vi "Debug Dequeuer.vi"() -> ()   [LabVIEW 2013]
panel:
  out "Waveform Chart":dbl[][](graph)
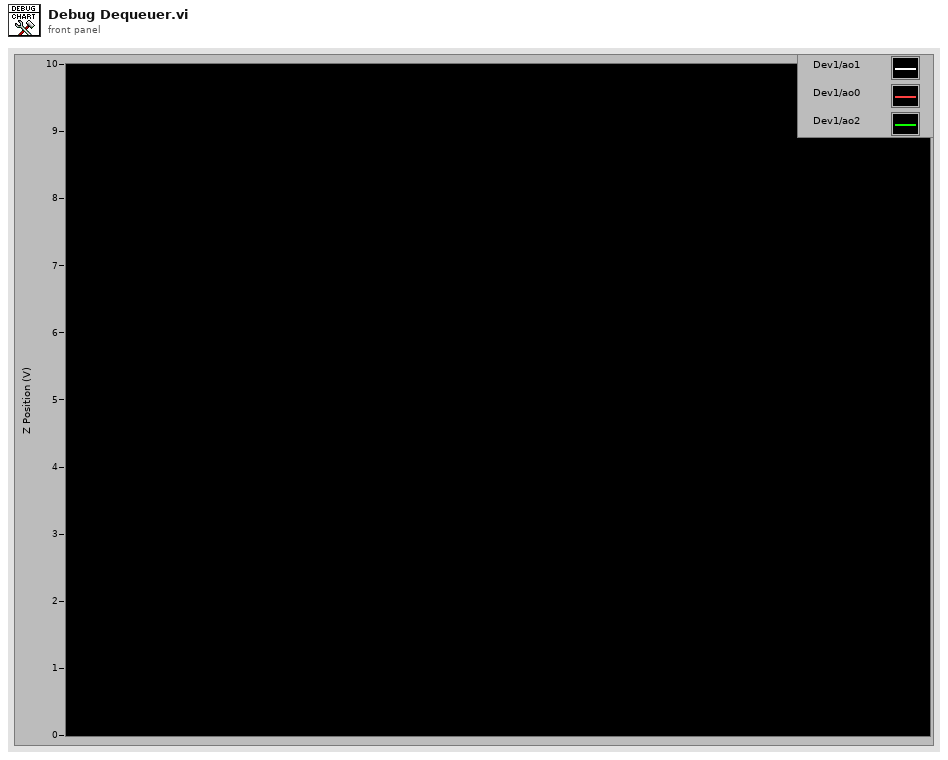
[diagram p1: front panel]
types:
  T1 = typedef "Sidecar Debug Queue.ctl" = refnum<queue>
  T2 = typedef "Experimental Configuration.ctl" = cluster{"Output Waveforms":waveform(dbl)[], "Output Channels":string, "Input Channels":string, "Post-Hook Occurence":refnum<k4>}
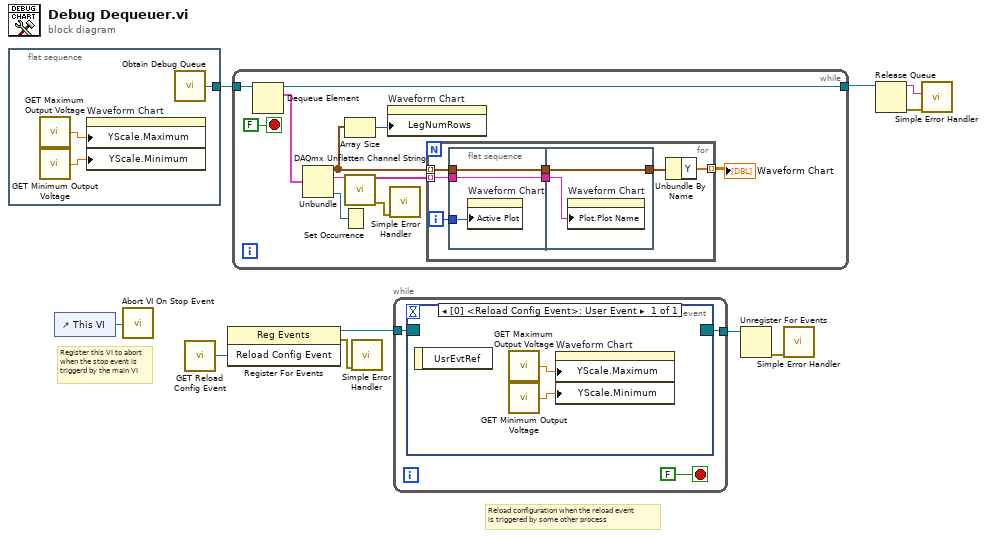
[diagram p0: block diagram]
diagram:
  # "Reload configuration when the reload event\nis triggered by some other process"
  # "Register this VI to abort\nwhen the stop event is\ntriggerd by the main VI"
  n1 = flat-sequence {
    tunnel: [w13] -> w10
    frame #0 {
      n2 = call "GET Maximum Output Voltage.vi"() -> ("Maximum Output Voltage"=w12:dbl)
      n3 = call "GET Minimum Output Voltage.vi"() -> ("Minimum Output Voltage"=w11:dbl)
      n4 = property on="Waveform Chart" class="WFChart (strict)"("YScale.Maximum"=w12, "YScale.Minimum"=w11) -> ()  [unwired: 2 in, 2 out]
      n5 = call "Obtain Debug Queue.vi"() -> ("Debug Queue"=w13:T1)
    }
  }
  n6 = control-ref of="This VI"() -> (w6:refnum<vi>)
  n7 = call "Abort VI On Stop Event.vi"("VI Reference"=w6) -> ()
  n8 = call "GET Reload Config Event.vi"() -> ("Reload Config Event"=w5:refnum<user-event>)
  n9 = register-events(w5) -> (reference out=w4:refnum<event-registration>, error out=w3:errorcluster)  [unwired: 2 in]
  n10 = while {
    tunnel: w10 -> [w23]
    tunnel: [w22] -> w9
    stop <- FALSE stop-if-true
    n11 = Dequeue Element(queue=w23) -> (queue out=w22:T1, element=w21:T2)  [unwired: 2 in, 2 out]
    n12 = Unbundle(w21) -> ("Output Waveforms"=w19:waveform(dbl)[], "Output Channels"=w17:string, "Post-Hook Occurence"=w20:refnum<k4>)  [unwired: 1 out]
    n13 = Set Occurrence(w20) -> ()
    n14 = Array Size(array=w19) -> (size(s)=w18:i32)
    n15 = call <vilib>:"DAQmx Unflatten Channel String.vi"("names in"=w17) -> ("names out"=w16:string[], "error out"=w15:errorcluster)  [unwired: 13 in]
    n16 = property on="Waveform Chart" class="WFChart (strict)"("LegNumRows"=w18) -> ()  [unwired: 2 in, 2 out]
    n17 = call <vilib>:"Simple Error Handler.vi"("error in (no error)"=w15) -> ()  [unwired: 4 in, 5 out]
    n18 = for {
      tunnel: w19 -> [w31] mode=indexing
      tunnel: w16 -> [w30] mode=indexing
      tunnel: [w25] -> w14 mode=indexing
      i -> [w29]
      n19 = flat-sequence {
        tunnel: w31 -> [w34]
        tunnel: w30 -> [w33]
        tunnel: w29 -> [w32]
        tunnel: [w34] -> w28
        tunnel: [w33] -> w27
        tunnel: w27 -> [w36]
        tunnel: w28 -> [w35]
        tunnel: [w35] -> w26
        frame #0 {
          n20 = property on="Waveform Chart" class="WFChart (strict)"("Active Plot"=w32) -> ()  [unwired: 2 in, 2 out]
        }
        frame #1 {
          n21 = property on="Waveform Chart" class="WFChart (strict)"("Plot.Plot Name"=w36) -> ()  [unwired: 2 in, 2 out]
        }
      }
      n22 = Unbundle By Name(w26) -> ("Y"=w25:dbl[])
    }
    "Waveform Chart" <- w14
  }
  n23 = call <vilib>:"Simple Error Handler.vi"("error in (no error)"=w3) -> ()  [unwired: 4 in, 5 out]
  n24 = while {
    tunnel: [w39] -> w2
    tunnel: w4 -> [w38]
    stop <- FALSE stop-if-true
    n25 = event shown="[0] <Reload Config Event>: User Event" {
      selector: w38 -> [_]
      dyn-events: [_] -> w39
      timeout: _ -> [_]
      event User Event {
        n26 = event-data() -> ()  [unwired: 1 in, 1 out]
        n27 = call "GET Maximum Output Voltage.vi"() -> ("Maximum Output Voltage"=w40:dbl)
        n28 = call "GET Minimum Output Voltage.vi"() -> ("Minimum Output Voltage"=w41:dbl)
        n29 = property on="Waveform Chart" class="WFChart (strict)"("YScale.Maximum"=w40, "YScale.Minimum"=w41) -> ()  [unwired: 2 in, 2 out]
      }
    }
  }
  n30 = Unregister For Events(event registration refnum=w2) -> (error out=w1:errorcluster)  [unwired: 1 in]
  n31 = call <vilib>:"Simple Error Handler.vi"("error in (no error)"=w1) -> ()  [unwired: 4 in, 5 out]
  n32 = Release Queue(queue=w9) -> (queue name=w8:string, error out=w7:errorcluster)  [unwired: 2 in, 1 out]
  n33 = call <vilib>:"Simple Error Handler.vi"("error source (\" \")"=w8, "error in (no error)"=w7) -> ()  [unwired: 3 in, 5 out]
